vi "U8ArrayToStr(cast).vi"(1 "U8数组":u8[](array[numeric]) format="%.0x") -> (0 "字符串":string)   [LabVIEW 2012]
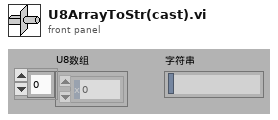
[diagram p1: front panel]
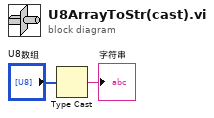
[diagram p0: block diagram]
diagram:
  n1 = Type Cast(x="U8数组") -> (*(type *) &x=→"字符串":string)  [unwired: 1 in]
